vi "ActTurn.vi"(9 "FirstTime":bool, 10 "MaxSpeed (ft/s)":dbl, 11 "Degrees":dbl) -> (0 "RightSpeedDemand":dbl, 1 "LeftSpeedDemand":dbl, 2 "Unfiltetred Done":bool, 3 "Done":bool)   [LabVIEW 2020]
doc: "Drive the robot straight in arcade drive\nList of things to tune:\n-MaxSpeed\n-ErrorThresh\n-ErrorDead\n-MinOutput\n-MaxOutput\n-Count\n\nInputs:\n--Dist -- Double -- in dwegrees\n-- MaxSpeed -- Double -- in ft/s, the MaxSpeed the robot can go (NEEDS TO BE TUNED)\n-- First Time - Bool -- is this the first time the distance is changing? \n\nOutputs:\n-- Done -- Bool -- has the robot reached its target distance\n-- Unfilt. L Target -- Bool -- unfilteredOnTarget for Left, for debugging purposes\n-- Unfilt. R Target -- Bool -- unfilteredOnTarget for Right, for debugging purposes"
uses:
  <vilib>/Rock Robotics/WPI/ThirdParty/JAS_Junk/TrajLib/Trajectory_Library.lvlib
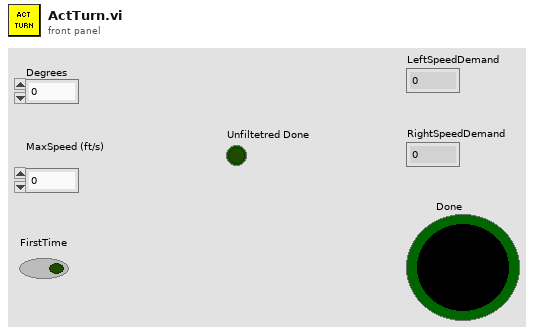
[diagram p1: front panel]
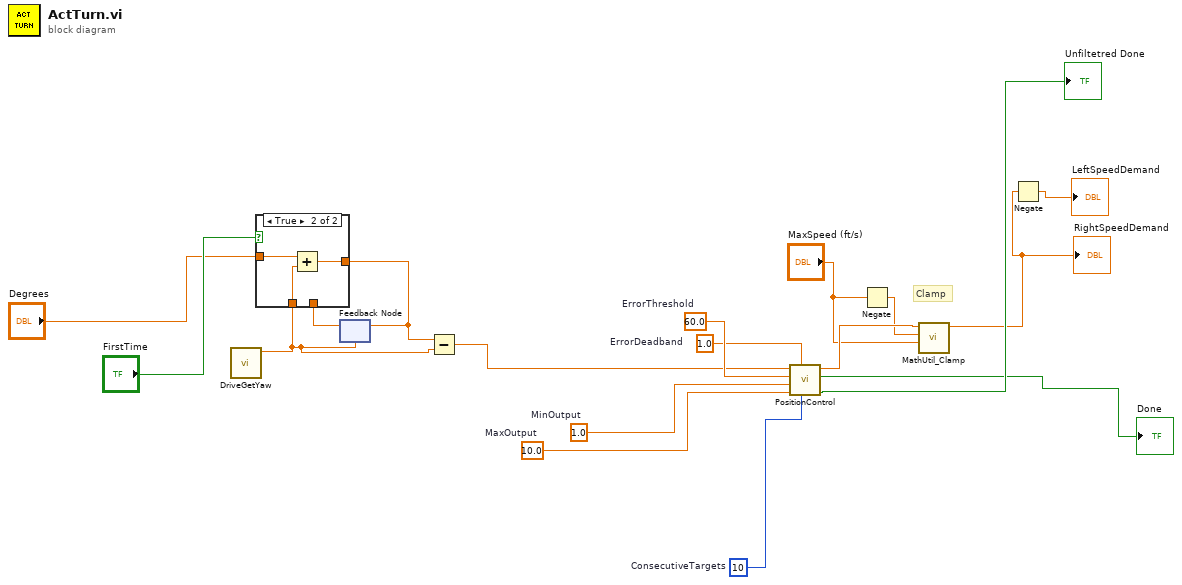
[diagram p0: block diagram]
diagram:
  w7 = 10.0  # MaxOutput
  w8 = 1.0  # MinOutput
  w13 = 10  # ConsecutiveTargets
  w14 = 1.0  # ErrorDeadband
  w15 = 60.0  # ErrorThreshold
  # "Clamp"
  n1 = call "DriveGetYaw.vi"() -> ("Yaw"=w3:dbl)  [unwired: 11 in]
  n2 = feedback #1(w3) -> (w16:dbl)
  n3 = case shown="True" "FirstTime" {
    tunnel: "Degrees" -> [_ w22]
    tunnel: [w19 w21] -> w9
    tunnel: w16 -> [w19 _]
    tunnel: w3 -> [_ w20]
    frame False {
    }
    frame True {
      n4 = Add(x=w22, y=w20) -> (x+y=w21:dbl)
    }
  }
  n5 = feedback-in #1(w9) -> ()
  n6 = Subtract(x=w9, y=w3) -> (x-y=w6:dbl)
  n7 = call "PositionControl.vi"("ConsecutiveTargets"=w13, "ErrorDeadband"=w14, "MaxOutput"=w7, "MinOutput"=w8, "ErrorThreshold"=w15, "Error"=w6) -> ("UnfilteredOnTarget"=→"Unfiltetred Done":bool, "OnTarget"=→"Done":bool, "OutputValue"=w12:dbl)  [unwired: 3 in]
  n8 = Negate(x="MaxSpeed (ft/s)") -> (-x=w11:dbl)
  n9 = call <vilib>:"MathUtil_Clamp.vi"("High Limit"="MaxSpeed (ft/s)", "Low Limit"=w11, "Value"=w12) -> ("Result"=w1:dbl)  [unwired: 8 in]
  "RightSpeedDemand" <- w1
  n10 = Negate(x=w1) -> (-x=→"LeftSpeedDemand":dbl)
